vi "Configure Reference Time Base.vi"(8 "error in (no error)":errorcluster, 10 "External ref. enable (True)":bool=TRUE, 11 "VISA resource name":refnum<visa-resource-name>) -> (0 "error out":errorcluster, 3 "VISA resource name out":refnum<visa-resource-name>)   [LabVIEW 2020, in "Counter.lvlib" / "PICOTEST U62XXA series.lvlib"]
doc: "Configures the Reference Time base to use an external signal instead of the default internal signal. If this external signal is not valid, an error is generated. Also, once a valild signal is connected to the External reference port, the counter automatically uses that signal.\n\n<B>Note:</B>\n\nFor the <B>U6200A and U6220A</B>, the External reference Only <B>10MHz</B> is valid for the <B>U6200A and U6220A</B>."
uses:
  PICOTEST U62XXA series.lvlib
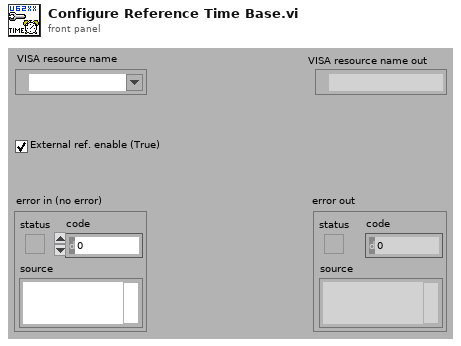
[diagram p1: front panel]
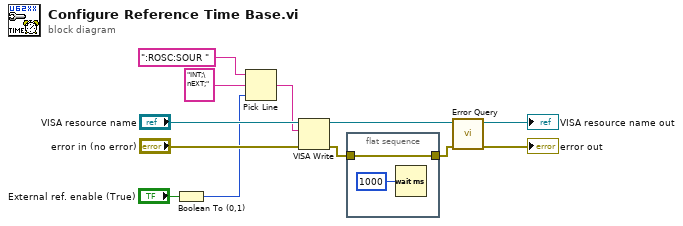
[diagram p0: block diagram]
diagram:
  n1 = Boolean To (0,1)(Boolean="External ref. enable (True)") -> (0, 1=w3:i16)
  n2 = Pick Line(string ("")=":ROSC:SOUR ", multi-line string="INT;\nEXT;", line index=w3) -> (output string=w7:string)
  n3 = VISA Write(VISA resource name="VISA resource name", write buffer=w7, error in (no error)="error in (no error)") -> (VISA resource name out=w11:refnum<visa-resource-name>, error out=w2:errorcluster)  [unwired: 1 out]
  n4 = flat-sequence {
    tunnel: w2 -> [w14]
    tunnel: [w14] -> w1
    frame #0 {
      n5 = Wait (ms)(milliseconds to wait=u32 1000) -> ()  [unwired: 1 out]
    }
  }
  n6 = call "Error Query.vi"("error in (no error)"=w1, "VISA resource name"=w11) -> ("error out"=→"error out":errorcluster, "VISA resource name out"=→"VISA resource name out":refnum<visa-resource-name>)  [unwired: 6 in, 2 out]
